vi "Write 2D Array to TDMS Log File.vi"(8 "error in (no error)":errorcluster, 10 "TDMS Write 2D Array Parameters":T1) -> (0 "error out":errorcluster)   [LabVIEW 2025, in "Data Logger v2.lvlib"]
doc: "Writes a 2D array to the TDMS log file.\n_____\nCreated using Delacor QMH Event Scripter 5.0.0.112."
uses:
  Data Logger v2.lvlib
  Write TDMS 2D Array Parameters--cluster.ctl
  Write 2D Array to TDMS Log File Argument--cluster.ctl
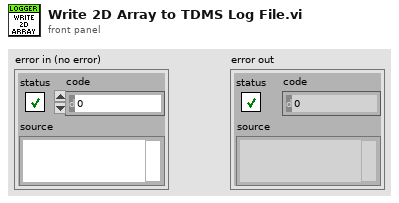
[diagram p1: front panel]
types:
  T1 = typedef "Data Logger v2.lvlib/Write TDMS 2D Array Parameters--cluster.ctl" = cluster{"Group":string, "Channel Names":string[], "Data":dbl[][]}
  T2 = typedef "Data Logger v2.lvlib/Write 2D Array to TDMS Log File Argument--cluster.ctl" = cluster{"TDMS Write 2D Array Parameters":T1}
  T3 = typedef "Data Logger v2.lvlib/Request Events--cluster.ctl" = cluster{"Stop Module":refnum<user-event>, "Show Panel":refnum<user-event>, "Hide Panel":refnum<user-event>, "Get Module Execution Status":refnum<user-event>, "Show Diagram":refnum<user-event>, "Change Panel":refnum<user-event>, "Create New TDMS Log File":refnum<user-event>, "Write 2D Array to TDMS Log File":refnum<user-event>, "Close TDMS File":refnum<user-event>, "Write TDMS 2D String Array":refnum<user-event>, "Set Root Folder Path":refnum<user-event>, "Create New TDMS Log File (Relative Path)":refnum<user-event>, "Set Properties":refnum<user-event>}
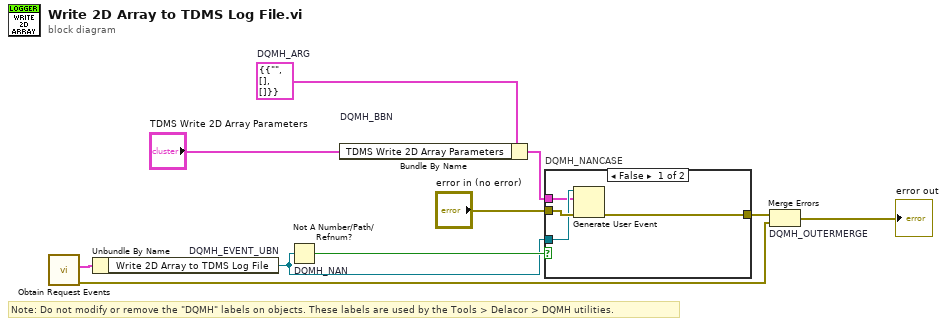
[diagram p0: block diagram]
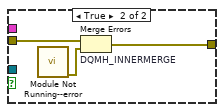
[diagram p2: hidden frame]
diagram:
  w4 = T2 {"TDMS Write 2D Array Parameters"={"Group"="", "Channel Names"=[], "Data"=[]}}  # DQMH_ARG
  # "Note: Do not modify or remove the \"DQMH\" labels on objects. These labels are used by the Tools > Delacor > DQMH utilities."
  n1 = call "Obtain Request Events.vi"() -> ("error out"=w2:errorcluster, "Data Logger v2 Request Events"=w1:T3)  [unwired: 10 in]
  n2 = Unbundle By Name "DQMH_EVENT_UBN"(w1) -> ("Write 2D Array to TDMS Log File"=w6:refnum<user-event>)
  n3 = Not A Number/Path/Refnum? "DQMH_NAN"(number/path/refnum=w6) -> (NaN/Path/Refnum?=w7:bool)
  n4 = Bundle By Name "DQMH_BBN"(cluster=w4, "TDMS Write 2D Array Parameters"="TDMS Write 2D Array Parameters") -> (w8:T2)
  n5 = case "DQMH_NANCASE" shown="False" w7 {
    tunnel: "error in (no error)" -> [w14 w17]
    tunnel: [w13 w16] -> w5
    tunnel: w6 -> [w12 _]
    tunnel: w8 -> [w11 _]
    frame False {
      n6 = Generate User Event(user event=w12, event data cluster=w11, error in=w14) -> (error out=w13:errorcluster)  [unwired: 1 in, 1 out]
    }
    frame True {
      n7 = call "Module Not Running--error.vi"() -> ("error out"=w15:errorcluster)  [unwired: 11 in]
      n8 = Merge Errors "DQMH_INNERMERGE"(w17, w15) -> (w16:errorcluster)
    }
  }
  n9 = Merge Errors "DQMH_OUTERMERGE"(w5, w2) -> (→"error out":errorcluster)
